vi "from string.vi"(8 "error in":errorcluster, 9 "data":string, 10 "version":string, 11 "tag bus configurable plugin module configuration in":refnum<class "tag bus processing plugin module configuration.lvclass">) -> (0 "error out":errorcluster, 3 "tag bus configurable plugin module configuration out":refnum<class "tag bus processing plugin module configuration.lvclass">)   [LabVIEW 2013, in "tag bus processing plugin module configuration.lvclass"]
doc: "Provides an interface for loading a module configuration from a file or other serialized data source. It is recommended that all children of this class store data in two sets--data required for its own initialization, and any data required for parent initialization--and that each implementation uses the <b>Call Parent Method</b> primitive to de-serialize parent information. As a result, it is expected that every module configuration class calls <b>component configuration.lvclass:From String.vi</b>."
uses:
  tag bus processing plugin module configuration.lvclass
  <vilib>/NI/Tag Bus Module Framework/module configuration/TBM module configuration.lvclass
  processing channels.ctl
  <vilib>/NI/Tag Bus Module Framework/channel/TBM channel.lvclass
  tag bus processing plugin module configuration.lvclass/tag bus processing plugin module configuration.ctl
  <vilib>/NI/Tag Bus Module Framework/root configuration/wrap data.vi
  <vilib>/NI/Tag Bus Module Framework/root configuration/create GUID.vi
  <vilib>/NI/Tag Bus Module Framework/root configuration/TBM configuration.lvclass
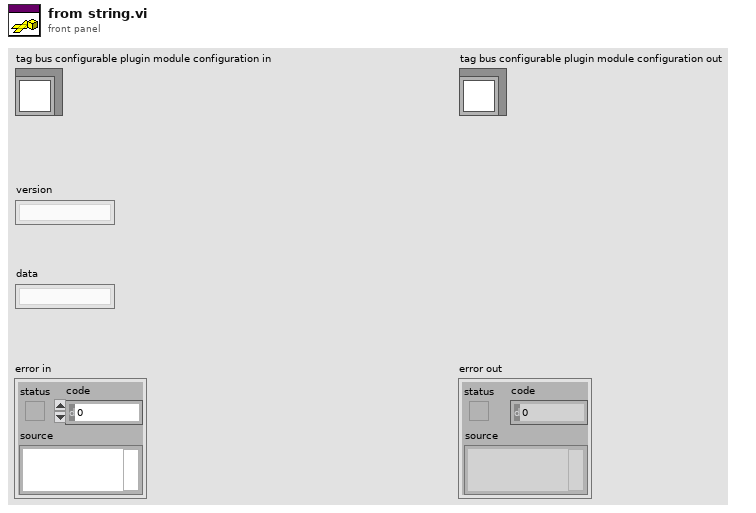
[diagram p1: front panel]
types:
  T1 = typedef "tag bus processing plugin module configuration.lvclass/processing channels.ctl" = cluster{"parameter":refnum<class "TBM channel.lvclass">, "result":refnum<class "TBM channel.lvclass">}
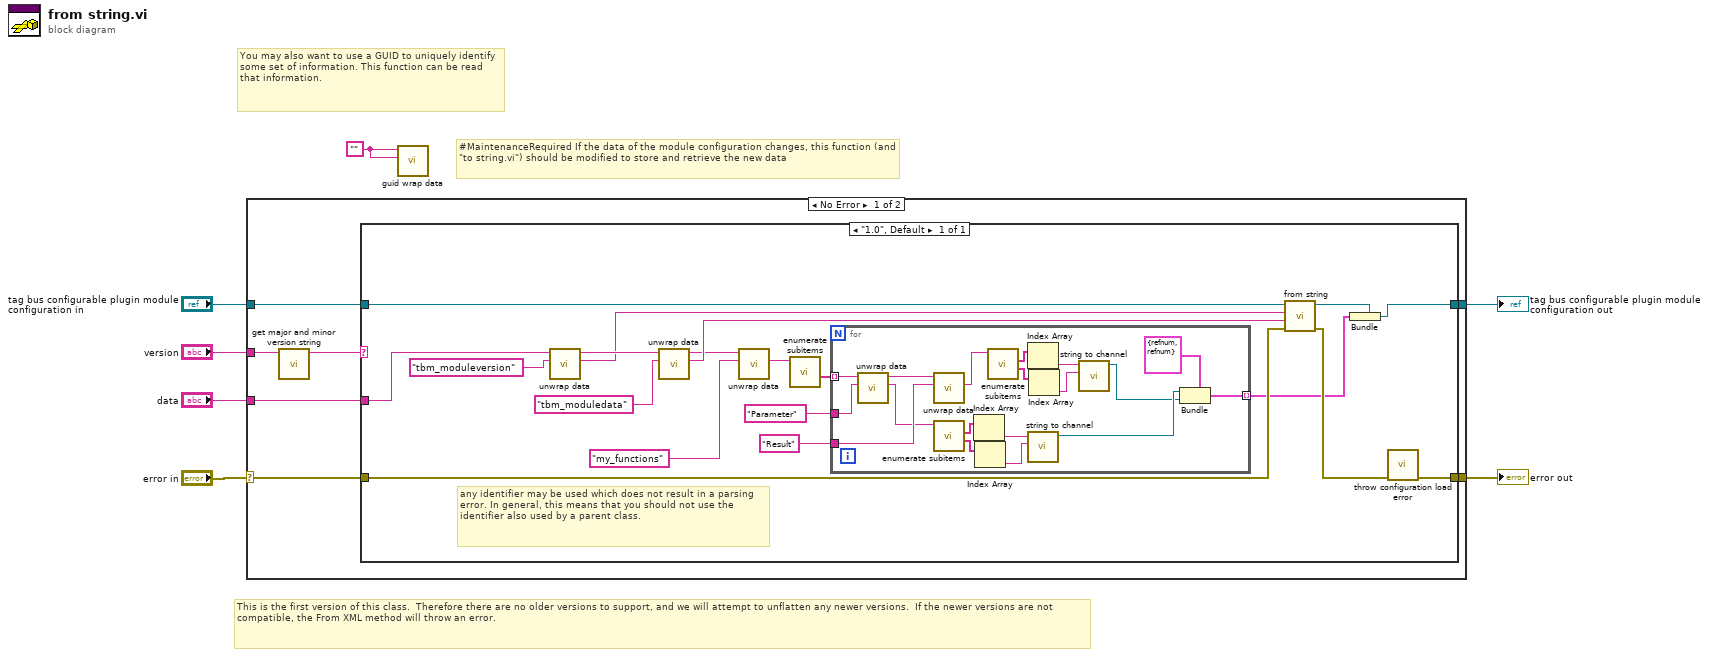
[diagram p0: block diagram]
diagram:
  w7 = ""
  # "You may also want to use a GUID to uniquely identify some set of information. This function can be read that information."
  # "#MaintenanceRequired If the data of the module configuration changes, this function (and \"to string.vi\") should be modified to store and retrieve the new data"
  # "This is the first version of this class.  Therefore there are no older versions to support, and we will attempt to unflatten any newer versions.  If the newer versions are not compatible, the From XML method will throw an error."
  n1 = case shown="No Error" "error in" {
    selector: "error in" -> [w8 w53]
    tunnel: "data" -> [w14 _]
    tunnel: "tag bus configurable plugin module configuration in" -> [w13 w52]
    tunnel: [w12 w52] -> w2
    tunnel: [w11 w53] -> w1
    tunnel: "version" -> [w10 _]
    frame No Error {
      n2 = call <vilib>:"get major and minor version string.vi"("full version"=w10) -> ("major.minor version"=w9:string)  [unwired: 10 in]
      n3 = case shown="\"1.0\", Default" w9 {
        tunnel: w14 -> [w29]
        tunnel: w8 -> [w28]
        tunnel: w13 -> [w33]
        tunnel: [w23] -> w12
        tunnel: [w31] -> w11
        frame "1.0", Default {
          # "any identifier may be used which does not result in a parsing error. In general, this means that you should not use the identifier also used by a parent class."
          n4 = call <vilib>:"unwrap data.vi"("identifier"="tbm_moduleversion" ("additional identifier"), "data to unwrap"=w29) -> ("unwrapped data"=w24:string, "remaining string"=w30:string)  [unwired: 8 in]
          n5 = call <vilib>:"unwrap data.vi"("identifier"="tbm_moduledata" ("additional identifier"), "data to unwrap"=w30) -> ("unwrapped data"=w26:string, "remaining string"=w22:string)  [unwired: 8 in]
          n6 = call <vilib>:"unwrap data.vi"("identifier"="my_functions" ("additional identifier"), "data to unwrap"=w22) -> ("unwrapped data"=w19:string)  [unwired: 8 in, 1 out]
          n7 = call <vilib>:"enumerate subitems.vi"("data to enumerate"=w19) -> ("associated data"=w18:string[])  [unwired: 8 in, 2 out]
          n8 = for {
            tunnel: w18 -> [w51] mode=indexing
            tunnel: "Parameter" ("identifier") -> [w50]
            tunnel: "Result" ("identifier") -> [w48]
            tunnel: [w34] -> w15 mode=indexing
            n9 = call <vilib>:"unwrap data.vi"("identifier"=w50, "data to unwrap"=w51) -> ("unwrapped data"=w47:string, "remaining string"=w49:string)  [unwired: 8 in]
            n10 = call <vilib>:"unwrap data.vi"("identifier"=w48, "data to unwrap"=w49) -> ("unwrapped data"=w42:string)  [unwired: 8 in, 1 out]
            n11 = call <vilib>:"enumerate subitems.vi"("data to enumerate"=w47) -> ("associated data"=w45:string[], "discovered subitems"=w46:string[])  [unwired: 8 in, 1 out]
            n12 = Index Array(array=w46) -> (element=w41:string)  [unwired: 1 in]
            n13 = Index Array(array=w45) -> (element=w40:string)  [unwired: 1 in]
            n14 = call <vilib>:"enumerate subitems.vi"("data to enumerate"=w42) -> ("associated data"=w44:string[], "discovered subitems"=w43:string[])  [unwired: 8 in, 1 out]
            n15 = Index Array(array=w43) -> (element=w38:string)  [unwired: 1 in]
            n16 = call <vilib>:"string to channel.vi"("channel data"=w40, "identifier"=w41) -> ("channel in"=w36:refnum<class "TBM channel.lvclass">)  [unwired: 9 in]
            n17 = Index Array(array=w44) -> (element=w39:string)  [unwired: 1 in]
            n18 = call <vilib>:"string to channel.vi"("channel data"=w39, "identifier"=w38) -> ("channel in"=w35:refnum<class "TBM channel.lvclass">)  [unwired: 9 in]
            n19 = Bundle(cluster=T1 {"parameter"=refnum, "result"=refnum} ("processing cluster"), "parameter"=w36, "result"=w35) -> (w34:T1)
          }
          n20 = call-parent "from string.vi"("error in"=w28, "data"=w26, "version"=w24, "module configuration in"=w33) -> ("error out"=w20:errorcluster, "module configuration out"=w32:refnum<class "tag bus processing plugin module configuration.lvclass">)  [unwired: 6 in]
          n21 = Bundle(cluster=w32, w15) -> (w23:refnum<class "tag bus processing plugin module configuration.lvclass">)
          n22 = call <vilib>:"throw configuration load error.vi"("error in"=w20) -> ("error out"=w31:errorcluster)  [unwired: 10 in]
        }
      }
    }
    frame Error {
    }
  }
  "error out" <- w1
  "tag bus configurable plugin module configuration out" <- w2
  n23 = call <vilib>:"guid wrap data.vi"("identifier"=w7, "data to wrap"=w7) -> ()  [unwired: 8 in, 2 out]
